vi "Dashboard Main.vi"() -> ()   [LabVIEW 2015]
uses:
  <vilib>/Utility/miscctls.llb/LVRowAndColumnTypeDef.ctl
  <vilib>/event_ctls.llb/eventvkey.ctl
  <vilib>/Rock Robotics/WPI/Dashboard/WPI_DashboardLogging Global.vi
  <vilib>/Rock Robotics/Network Tables/NT Read Numeric Array.vi
  <vilib>/Utility/config.llb/Write Key (String).vi
  <vilib>/Utility/config.llb/Write Key (I32).vi
  <vilib>/Utility/config.llb/NI_LVConfig.lvlib
panel:
  in  "Stop":bool
  in  "TCP":refnum<k5>
  in  "Rec Mode":enum32{"Stop", "Record", "Playback"}(radio)
  in  "Vision":u16(ring) items=["Camera Off", "USB Camera SW", "USB Camera HW", "IP Camera"]
  out "Camera IP":string
  out "Image Message":string="Timeout in Camera Communications"
  in  "Dashboard Tab":T1(tab)
  out "NT Connected":bool
  in  "Camera Settings":T2={"Frame Rate"=30, "Compression"=30, "Size"=1} {"Frame Rate" scale=1.0..30.0; "Size" items=["640x480", "320x240", "160x120"]}
  out "MotorChart R":cluster{"Numeric":dbl, "Numeric":dbl}(graph)
  out "MotorChart L":T3(graph)
  out "MotorSliders R":cluster{"MotorSlide1":dbl, "MotorSlide2":dbl} {"MotorSlide2" scale=-1.0..1.0 scale format="%#_2e"; "MotorSlide1" scale=-1.0..1.0 scale format="%#_2e"}
  out "MotorSliders L":T4 {"MotorSlide4 2" scale=0.0..14.0 scale format="%#_2e"; "MotorSlide2" scale=-1.0..1.0 scale format="%#_2e"; "MotorSlide1" scale=-1.0..1.0 scale format="%#_2e"}
  out "Gyro":dbl(knob) scale=0.0..360.0
  out "JS1 Z":dbl(slide) scale=-1.0..1.0 scale format="%#_2e"
  out "JS1 Graph":cluster{"X":dbl, "Y":dbl}[](graph)
  out "JS1 Buttons":T5
  out "JS2 Z":dbl(slide) scale=-1.0..1.0 scale format="%#_2e"
  out "JS2 Graph":cluster{"X":dbl, "Y":dbl}[](graph)
  out "JS2 Buttons":T5
  out "Mode":T6(ring)=enum."Auto Disabled"
  in  "DB Camera Config":bool
  out "fps":dbl format="%#.1g"
  out "Mbps":dbl format="%#.1g"
  out "Mbps 2":bool
  in  "DB/String 9":string
  in  "DB/String 8":string
  in  "DB/String 7":string
  in  "DB/String 6":string
  in  "DB/String 5":string
  in  "DB/String 4":string
  in  "DB/String 3":string
  in  "DB/String 2":string
  in  "DB/String 1":string
  in  "DB/String 0":string
  in  "DB/Slider 0":dbl(slide) scale=0.0..5.0
  in  "DB/Slider 1":dbl(slide) scale=0.0..5.0
  in  "DB/Slider 2":dbl(slide) scale=0.0..5.0
  in  "DB/Slider 3":dbl(slide) scale=0.0..5.0
  out "DB/LED 3":bool
  out "DB/LED 2":bool
  out "DB/LED 1":bool
  out "DB/LED 0":bool
  in  "DB/Button 3":bool
  in  "DB/Button 2":bool
  in  "DB/Button 1":bool
  in  "DB/Button 0":bool caption="New Name"
  out "Data AQ - Y axis":dbl(graph)
  out "Turn Power":dbl
  out "Throttle":dbl
  in  "Ka":dbl
  in  "Kv":dbl=0.08333
  in  "Max Acceleration":dbl=8.0
  in  "Max Velocity":dbl=13.5
  in  "Drive Distance":dbl
  in  "Test Slider":dbl(slide) scale=0.0..100.0 scale format="%#_3g"
  in  "On/Off":bool caption="Solenoid"
  in  "Test Name":u16(ring) items=["Select the test to run..."]
  in  "Test Tree":string(tree)
  in  "Motor":cluster{"Value":dbl, "Enable":bool} {"Value" scale=-1.0..1.0 scale format="%#_3g"}
  out "Progress":T7 {"Test Progress" scale=0.0..100.0}
  in  "Rev/Fwd":cluster{"Forward":bool, "Reverse":bool}
  in  "Test Ring":u16(ring) items=["Monochrome", "Color"]
  out "Cmd Status":string
  in  "Execute Command":bool
  in  "Command Params":string[][](table)
  in  "Command Selection":i32(listbox)
  in  "CheckList":i32(listbox)
  out "Tree":string(tree)
  out "Camera Image":T8(plugin-control)
  out "Boolean":bool
  # "Left"
  # "Front"
  # "Right"
  # "Battery"
  # "This tab is a great place for autonomous settings and robot-specific values.\nPlace controls and indicators inside this tab and match name to\nDashboard Variables on robot. You can also delete this comment."
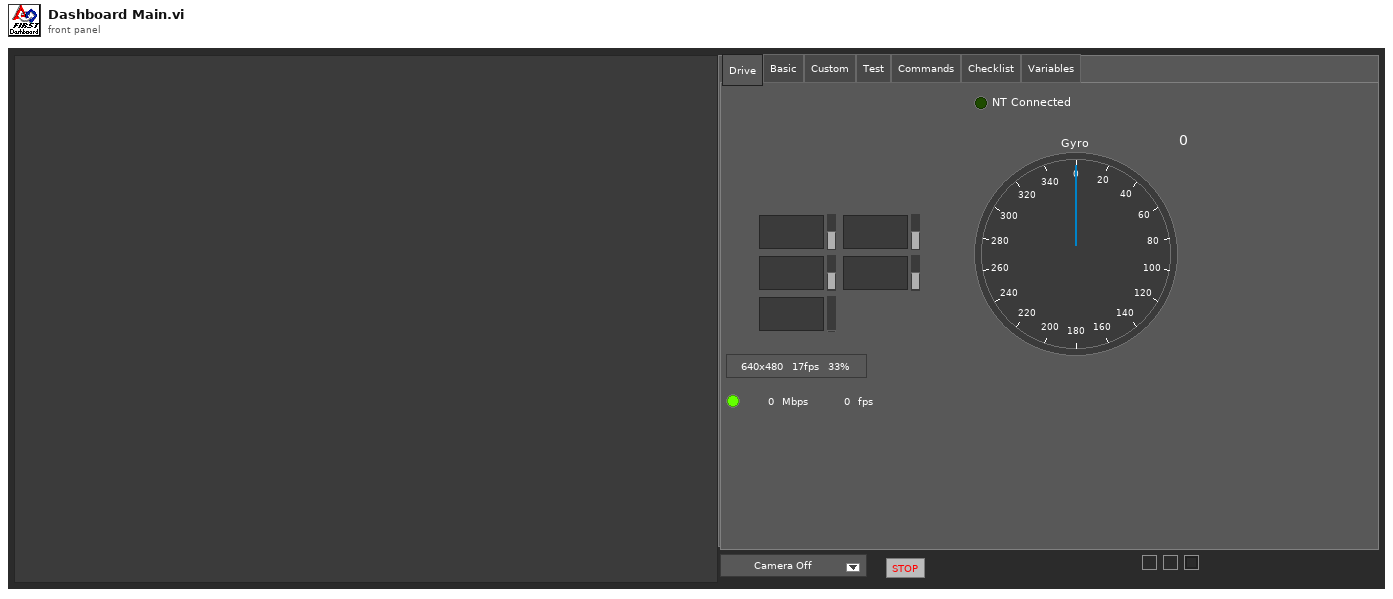
[diagram p1: front panel]
types:
  T1 = enum32{"Drive", "Basic", "Custom", "Test", "Commands", "Checklist", "Variables"}
  T2 = cluster{"Frame Rate":i32, "Compression":i32, "Size":u16}
  T3 = cluster{"Numeric":dbl, "Numeric":dbl, "Battery V":dbl}
  T4 = cluster{"MotorSlide1":dbl, "MotorSlide2":dbl, "MotorSlide4 2":dbl}
  T5 = cluster{bool, bool, bool, bool, bool, bool, bool, bool, bool, bool, bool, bool}
  T6 = enum8{"Tele-Op Disabled", "Tele-Op Enabled", "Auto Disabled", "Auto Enabled", "Test Disabled", "Test Enabled", "Disconnected", "No Code", "E-Stop"}
  T7 = cluster{"Test Progress":u8, "Test Progress Text":string}
  T8 = typedef "IMAQ Image.ctl" = refnum<image>
  T9 = cluster{"IDs":cluster{"RPC field ID":u16, "Unique ID":u16}, "String":string}
  T10 = enum32{"Drive", "Basic", "Custom", "Test", "Checklist", "Variables"}
  T11 = typedef "Image Type" = u32
  T12 = cluster{"Camera Image":refnum<vi>, "Dashboard Tab":refnum<vi>, "Boolean":refnum<vi>, "Vision":refnum<vi>, "Rec Mode":refnum<vi>, "Test Slider":refnum<vi>, "On/Off ":refnum<vi>, "Test Ring":refnum<vi>, "Rev/Fwd":refnum<vi>, "Test Name":refnum<vi>, "Motor":refnum<vi>, "Progress":refnum<vi>, "CheckList":refnum<vi>, "Tree":refnum<vi>, "Test Tree":refnum<vi>, "Command Params":refnum<vi>, "Command Selection":refnum<vi>, "Execute Command":refnum<vi>, "Cmd Status":refnum<vi>}
  T13 = cluster{"Error Strings":string, "Disable Counts":cluster{u16, u16}, "Rail Faults":cluster{u16, u16, u16}, "Robot IP":string, "DB Mode":u8, "Event Info":cluster{"Name":string, "Type":u8, "Number":u16, "Replay":u8}, "Camera Addr":string}
  T14 = cluster{"Storage":cluster{"Disk Free":u64, "RAM Block":u32, "RAM free":u32}, "CPU Utilization":cluster{"CPU % ISR":sgl, "CPU % Time Crit":sgl, "CPU % Timed Str":sgl, "CPU % High":sgl, "CPU % Above":sgl, "CPU % Normal":sgl, "CPU % Low":sgl}, "CAN":cluster{"% Bus Utilization":sgl, "Bus Off Cnt":u32, "TX_FIFO Full Cnt":u32, "Receive Error Cnt":u8, "Transmit Error Cnt":u8}, "HID":cluster{"HID Outputs":u32, "Rumble Low":u16, "Rumble High":u16}[]}
  T15 = cluster{"Status bits":cluster{"Test Mode":bool, "Autonomous":bool, "Enabled":bool, "Code Start":bool, "Brownout":bool, "Reserved 2":bool, "Reserved 3":bool, "E-Stop":bool}, "Code Trace":cluster{"Disabled":bool, "TeleOp":bool, "Auto":bool, "Test":bool}, "Controller Type":enum16{"unknown", "cRIO", "roboRio"}, "Code?":enum16{"unknown", "noCode", "code"}, "Battery V":dbl}
  T16 = cluster{"Control Bits":cluster{"TestMode":bool, "Autonomous":bool, "Enabled":bool, "FMS Present":bool, bool, bool, bool, "E-Stop":bool}, "Team Station ":u8, "Countdown":sgl, "Joystick Values":cluster{"Axes":dbl[], "Buttons":bool[], "POVs":i16[]}[]}
  T17 = cluster{"Axes":dbl[], "Buttons":bool[], "POVs":i16[]}[]
  T18 = cluster{"Axes":dbl[], "Buttons":bool[], "POVs":i16[]}
  T19 = cluster{"Buttons[0]":bool, "Buttons[1]":bool, "Buttons[2]":bool, "Buttons[3]":bool, "Buttons[4]":bool, "Buttons[5]":bool, "Buttons[6]":bool, "Buttons[7]":bool, "Buttons[8]":bool, "Buttons[9]":bool, "Buttons[10]":bool, "Buttons[11]":bool}
  T20 = typedef "NI_LVConfig.lvlib/Config Data RefNum.ctl" = refnum<k1>
  T21 = cluster{"Operation":enum16{"Update", "Clear"}, "Color Box":u32}[]
  T22 = typedef "eventvkey.ctl" = enum16{"ASCII", "Enter", "Return", "Shift", "Ctrl", "Alt", "Cmd", "Opt", "Caps", "NumLock", "Clear", "Break", "Up", "Down", "Left", "Right", "Insert", "Delete", "Home", "End", "PageUp", "PageDown", "Escape", "Help", "Pause", "ScrollLock", "F1", "F2", "F3", "F4", "F5", "F6", "F7", "F8", "F9", "F10", "F11", "F12", "F13", "F14", "F15", "F16", "F17", "F18", "F19", "F20", "F21", "F22", "F23", "F24", "Play", "VolumeUp", "VolumeDown", "Mute", "Two Byte Char"}
  T23 = cluster{"Image Size":bool, "Image Type":bool, "Pixel Value":bool, "ROI Information":bool, "Zoom Factor":bool}
  T24 = enum8{"Enabled", "Disabled", "Disabled and Grayed Out"}
  T25 = cluster{"Operation":enum16{"Update", "Clear"}, "Color Box":u32}
  T26 = typedef "LVRowAndColumnTypeDef.ctl" = cluster{"Row":i32, "Column":i32}
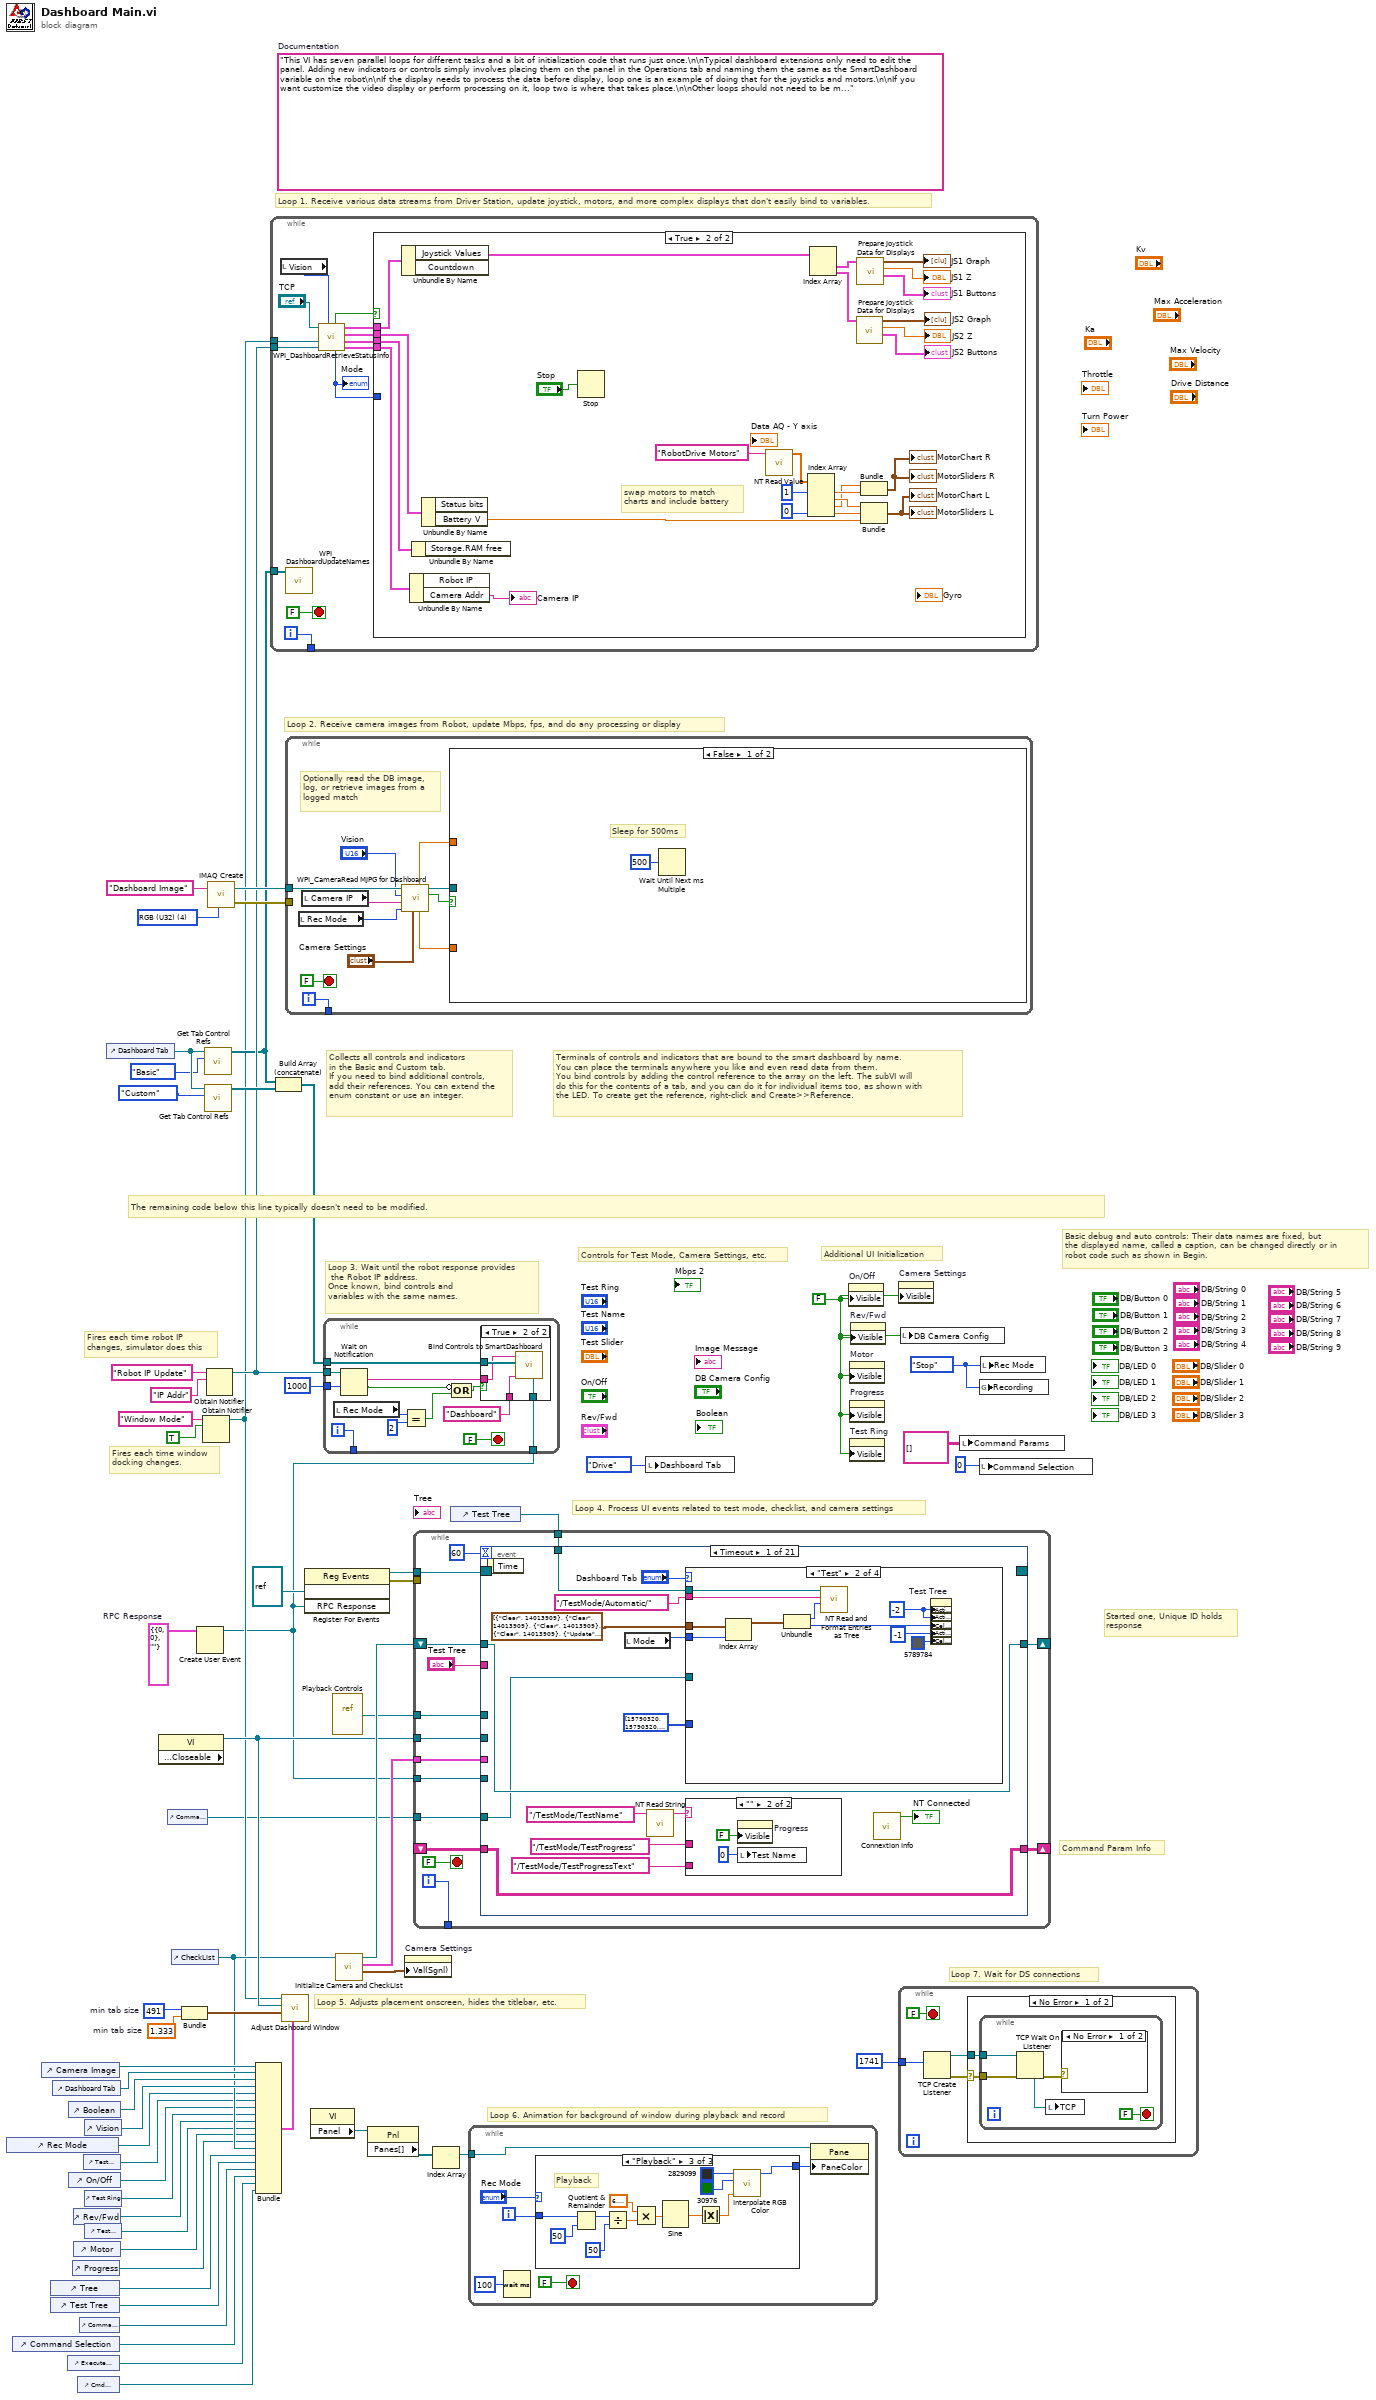
[diagram p0: block diagram]
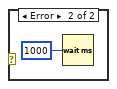
[diagram p2: hidden frame]
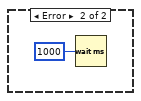
[diagram p3: hidden frame]
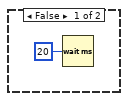
[diagram p4: hidden frame]
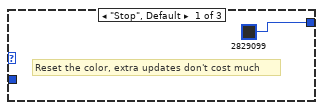
[diagram p5: hidden frame]
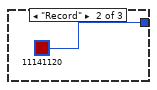
[diagram p6: hidden frame]
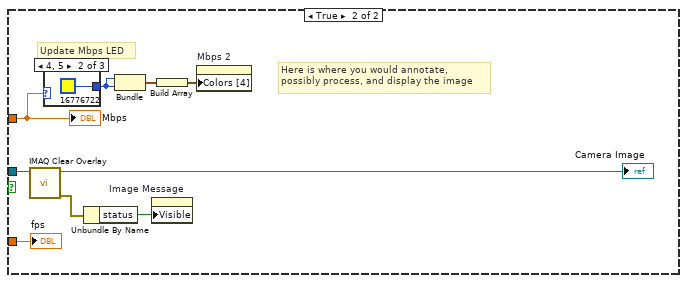
[diagram p8: hidden frame]
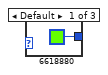
[diagram p9: hidden frame]
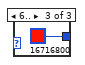
[diagram p10: hidden frame]
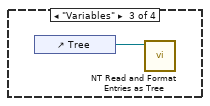
[diagram p12: hidden frame]
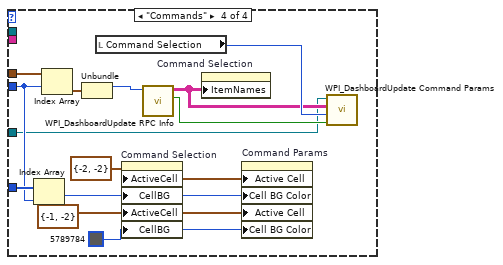
[diagram p13: hidden frame]
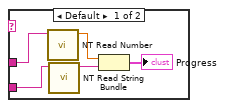
[diagram p14: hidden frame]
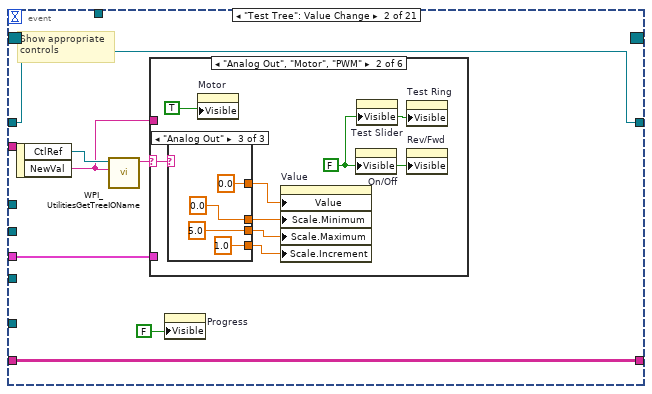
[diagram p15: hidden frame]
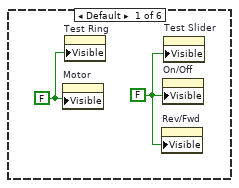
[diagram p16: hidden frame]
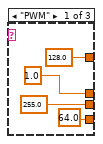
[diagram p17: hidden frame]
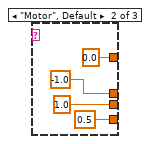
[diagram p18: hidden frame]
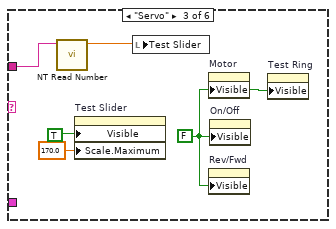
[diagram p19: hidden frame]
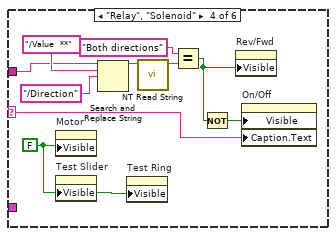
[diagram p20: hidden frame]
diagram:
  w7 = T9 {"IDs"={"RPC field ID"=0, "Unique ID"=0}, "String"=""}  # RPC Response
  w33 = 491  # min tab size
  w32 = 1.333  # min tab size
  w41 = enum32{"Stop", "Record", "Playback"}."Stop" ("Rec Mode")
  w15 = FALSE ("Visible")
  (unwired) "This VI has seven parallel loops for different tasks and a bit of initialization code that runs just once.\n\nTypical dashboard extensions only need to edit the panel. Adding new indicators or controls simply involves placing them on the panel in the Operations tab and naming them the same as the SmartDashboard variable on the robot\n\nIf the display needs to process the data before display, loop one is an example of doing that for the joysticks and motors.\n\nIf you want customize the video display or perform processing on it, loop two is where that takes place.\n\nOther loops should not need to be modified. They are pretty standard, and document the task they perform."  # Documentation
  w61 = T11 4 items=["Grayscale (U8)", "Grayscale (I16)", "Grayscale (SGL)", "Complex (CSG)", "RGB (U32)", "HSL (U32)", "RGB (U64)"] ("Image Type")
  # "Command Param Info"
  # "Started one, Unique ID holds\nresponse"
  # "Loop 7. Wait for DS connections"
  # "Basic debug and auto controls: Their data names are fixed, but\nthe displayed name, called a caption, can be changed directly or in\nrobot code such as shown in Begin."
  # "Controls for Test Mode, Camera Settings, etc."
  # "Additional UI Initialization"
  # "Loop 6. Animation for background of window during playback and record"
  # "Fires each time robot IP\nchanges, simulator does this"
  # "Fires each time window\ndocking changes."
  # "Collects all controls and indicators\nin the Basic and Custom tab.\nIf you need to bind additional controls,\nadd their references. You can extend the\nenum constant or use an integer."
  # "The remaining code below this line typically doesn't need to be modified."
  # "Loop 4. Process UI events related to test mode, checklist, and camera settings"
  # "Terminals of controls and indicators that are bound to the smart dashboard by name.\nYou can place the terminals anywhere you like and even read data from them.\nYou bind controls by adding the control reference to the array on the left. The subVI will\ndo this for the contents of a tab, and you can do it for individual items too, as shown with\nthe LED. To create get the reference, right-click and Create>>Reference."
  # "Loop 3. Wait until the robot response provides\n the Robot IP address.\nOnce known, bind controls and\nvariables with the same names."
  # "Loop 5. Adjusts placement onscreen, hides the titlebar, etc."
  # "Loop 1. Receive various data streams from Driver Station, update joystick, motors, and more complex displays that don't easily bind to variables."
  # "Loop 2. Receive camera images from Robot, update Mbps, fps, and do any processing or display"
  n1 = control-ref of="Rec Mode"() -> (w21:refnum<vi>)
  n2 = control-ref of="Command Selection"() -> (w6:refnum<vi>)
  n3 = control-ref of="Camera Image"() -> (w36:refnum<vi>)
  n4 = control-ref of="Tree"() -> (w25:refnum<vi>)
  n5 = control-ref of="Test Tree"() -> (w24:refnum<vi>)
  n6 = control-ref of="Dashboard Tab"() -> (w35:refnum<vi>)
  n7 = control-ref of="Execute Command"() -> (w8:refnum<vi>)
  n8 = control-ref of="Boolean"() -> (w30:refnum<vi>)
  n9 = control-ref of="On/Off"() -> (w19:refnum<vi>)
  n10 = control-ref of="Progress"() -> (w16:refnum<vi>)
  n11 = control-ref of="Rev/Fwd"() -> (w17:refnum<vi>)
  n12 = control-ref of="Motor"() -> (w22:refnum<vi>)
  n13 = control-ref of="Cmd Status"() -> (w2:refnum<vi>)
  n14 = control-ref of="Command Params"() -> (w9:refnum<vi>)
  n15 = control-ref of="Test Slider"() -> (w20:refnum<vi>)
  n16 = control-ref of="Vision"() -> (w34:refnum<vi>)
  n17 = control-ref of="Test Ring"() -> (w18:refnum<vi>)
  n18 = control-ref of="Test Name"() -> (w23:refnum<vi>)
  n19 = control-ref of="Dashboard Tab"() -> (w39:refnum<vi>)
  n20 = property class="VI" props=["Front Panel.Closeable"]() -> (reference out=w40:refnum<vi>)  [unwired: 2 in, 2 out]
  n21 = control-ref of="Command Params"() -> (w1:refnum<vi>)
  n22 = control-ref of="CheckList"() -> (w26:refnum<vi>)
  n23 = Bundle("min tab size"=w33, "min tab size"=w32) -> (w31:cluster{"min tab size":i32, "min tab size":dbl})  [unwired: 1 in]
  n24 = Create User Event(user event datatype=w7) -> (user event=w3:refnum<user-event>)  [unwired: 1 in, 1 out]
  n25 = Obtain Notifier(name (unnamed)="Window Mode", notification data type=TRUE) -> (notifier out=w12:refnum<notifier>)  [unwired: 2 in, 2 out]
  n26 = call <vilib>:"Get Tab Control Refs.vi"("Page Index"=T10."Basic" ("Dashboard Tab"), "TabControl in"=w39) -> ("ControlsOnPage"=w13:refnum<vi>[])  [unwired: 9 in]
  n27 = call <vilib>:"Get Tab Control Refs.vi"("Page Index"=T10."Custom" ("Dashboard Tab"), "TabControl in"=w39) -> ("ControlsOnPage"=w38:refnum<vi>[])  [unwired: 9 in]
  n28 = Obtain Notifier(name (unnamed)="Robot IP Update", notification data type="IP Addr" ("name (unnamed)")) -> (notifier out=w14:refnum<notifier>)  [unwired: 2 in, 2 out]
  n29 = call "IMAQ Create"("Image Name"="Dashboard Image", "Image Type"=w61) -> ("New Image"=w59:T8, "error out"=w58:errorcluster)  [unwired: 2 in, 1 out]
  n30 = Bundle("Camera Image"=w36, "Dashboard Tab"=w35, "Boolean"=w30, "Vision"=w34, "Rec Mode"=w21, "Test Slider"=w20, "On/Off"=w19, "Test Ring"=w18, "Rev/Fwd"=w17, "Test Name"=w23, "Motor"=w22, "Progress"=w16, "CheckList"=w26, "Tree"=w25, "Test Tree"=w24, "Command Params"=w9, "Command Selection"=w6, "Execute Command"=w8, "Cmd Status"=w2) -> (w27:T12)  [unwired: 1 in]
  n31 = while {
    tunnel: [w73] -> _
    tunnel: w14 -> [w67]
    tunnel: w13 -> [w66]
    tunnel: w12 -> [w62]
    i -> [w73]
    stop <- FALSE stop-if-true
    n32 = local read "Vision"() -> (w64:u16)
    n33 = call <vilib>:"WPI_DashboardUpdateNames.vi"("Controls on Tab"=w66) -> ()  [unwired: 11 in]
    n34 = call <vilib>:"WPI_DashboardRetrieveStatusInfo.vi"("Vision"=w64, "Binding Refnum"=w67, "Window Mode Notifier"=w62, "TCP Cnx"="TCP") -> ("Power and Errors"=w68:T13, "Robot Metrics"=w71:T14, "Status Info"=w72:T15, "Control Info"=w69:T16, "Robot Mode"=w65:T6, "Process?"=w70:bool)  [unwired: 2 in]
    "Mode" <- w65
    n35 = case shown="True" w70 {
      tunnel: w72 -> [_ w101]
      tunnel: w71 -> [_ w100]
      tunnel: w69 -> [_ w99]
      tunnel: w68 -> [_ w98]
      tunnel: w65 -> [_ _]
      frame False {
        n36 = Wait (ms)(milliseconds to wait=u32 20) -> ()  [unwired: 1 out]
      }
      frame True {
        # "swap motors to match\ncharts and include battery"
        n37 = Unbundle By Name(w99) -> ("Joystick Values"=w88:T17)  [unwired: 1 out]
        n38 = Unbundle By Name(w98) -> ("Camera Addr"=→"Camera IP":string)  [unwired: 1 out]
        n39 = Unbundle By Name(w100) -> ()  [unwired: 1 out]
        n40 = Unbundle By Name(w101) -> ("Battery V"=w89:dbl)  [unwired: 1 out]
        n41 = Stop(stop? (T)="Stop") -> ()
        n42 = call-poly <vilib>:"NT Read Value.vi"("Name"="RobotDrive Motors") -> ("Numeric Array"=w77:dbl[])  [unwired: 9 in, 1 out]
        n43 = Index Array(array=w77, index #1=1, index #4=0) -> (element #1=w93:dbl, element #2=w94:dbl, element #3=w92:dbl, element #4=w97:dbl)  [unwired: 2 in]
        n44 = Index Array(array=w88) -> (element #1=w87:T18, element #2=w82:T18)  [unwired: 2 in]
        n45 = call "Prepare Joystick Data for Displays.vi"("Joystick Values"=w82) -> ("Buttons"=→"JS2 Buttons":T19, "Z Axis"=→"JS2 Z":dbl, "Cartesian Data"=→"JS2 Graph":cluster{"X axis":dbl, "X axis":dbl}[])  [unwired: 8 in]
        n46 = call "Prepare Joystick Data for Displays.vi"("Joystick Values"=w87) -> ("Buttons"=→"JS1 Buttons":T19, "Z Axis"=→"JS1 Z":dbl, "Cartesian Data"=→"JS1 Graph":cluster{"X axis":dbl, "X axis":dbl}[])  [unwired: 8 in]
        n47 = Bundle("Numeric"=w92, "Numeric"=w93) -> (→"MotorChart R" →"MotorSliders R":cluster{"Numeric":dbl, "Numeric":dbl})  [unwired: 1 in]
        n48 = Bundle("Numeric"=w94, "Numeric"=w97, "Battery V"=w89) -> (→"MotorChart L" →"MotorSliders L":T3)  [unwired: 1 in]
      }
    }
  }
  n49 = Build Array (concatenate)(w13, w38) -> (w37:refnum<vi>[])
  n50 = call "Adjust Dashboard Window.vi"("Sizing Refnums"=w27, "Size Constraints"=w31, "VI"=w40, "WIn Mode"=w12) -> ()  [unwired: 8 in]
  n51 = while {
    tunnel: w59 -> [w110]
    tunnel: w58 -> [_]
    tunnel: [w111] -> _
    i -> [w111]
    stop <- FALSE stop-if-true
    # "Optionally read the DB image,\nlog, or retrieve images from a\nlogged match"
    n52 = local read "Rec Mode"() -> (w104:enum32{"Stop", "Record", "Playback"})
    n53 = local read "Camera IP"() -> (w102:string)
    n54 = call <vilib>:"WPI_CameraRead MJPG for Dashboard.vi"("Camera Settings"="Camera Settings", "Rec Mode"=w104, "Camera IP"=w102, "Camera Mode"="Vision", "Refnum in"=w110) -> ("Active"=w108:bool, "Refnum out"=w109:T8, "FPS"=w107:dbl, "Bandwidth (Mbps)"=w106:dbl)  [unwired: 3 in]
    n55 = case shown="False" w108 {
      tunnel: w109 -> [_ w117]
      tunnel: w106 -> [_ w116]
      tunnel: w107 -> [_ w114]
      frame False {
        # "Sleep for 500ms"
        n56 = Wait Until Next ms Multiple(millisecond multiple=u32 500) -> ()  [unwired: 1 out]
      }
      frame True {
        # "Here is where you would annotate,\npossibly process, and display the image"
        # "Update Mbps LED"
        n57 = call "IMAQ Clear Overlay"("Image"=w117) -> ("error out"=w121:errorcluster, "Image Out"=→"Camera Image":T8)  [unwired: 2 in, 7 out]
        n58 = case shown="4, 5" w116 {
          tunnel: [u32 6618880 ("Color Box") u32 16776722 ("Color Box") u32 16716800 ("Color Box")] -> w118
          frame Default {
          }
          frame 4, 5 {
          }
          frame 6.. {
          }
        }
        n59 = Unbundle By Name(w121) -> ("status"=w122:bool)
        n60 = Bundle("Color Box"=w118, "Color Box"=w118) -> (w120:cluster{"Color Box":u32, "Color Box":u32})  [unwired: 1 out]
        n61 = property on="Image Message" class="Str"("Visible"=w122) -> ()  [unwired: 2 in, 2 out]
        n62 = Build Array(w120) -> (w119:cluster{"Color Box":u32, "Color Box":u32}[])
        n63 = property on="Mbps 2" class="Bool (strict)"("Colors [4]"=w119) -> ()  [unwired: 2 in, 2 out]
        "Mbps" <- w116
        "fps" <- w114
      }
    }
  }
  n64 = register-events(refnum<vi> refnum, w3) -> (reference out=w45:refnum<event-registration>, error out=w44:errorcluster)  [unwired: 2 in]
  n65 = property class="VI"() -> ("Panel"=w48:refnum<vi>)  [unwired: 2 in, 2 out]
  n66 = while {
    tunnel: w37 -> [w138]
    tunnel: w14 -> [w136]
    tunnel: [w134] -> _
    tunnel: u32 1000 ("milliseconds to wait") -> [w133]
    tunnel: w3 -> [w126]
    i -> [w134]
    stop <- FALSE stop-if-true
    n67 = local read "Rec Mode"() -> (w129:enum32{"Stop", "Record", "Playback"})
    n68 = Wait on Notification(notifier=w136, timeout in ms (-1)=w133) -> (notification=w135:string, timed out?=w131:bool)  [unwired: 2 in, 2 out]
    n69 = Equal?(x=w129, y=u16 2 ("Rec Mode")) -> (x = y?=w130:bool)
    n70 = Compound Arithmetic op=OR(invert w131, w130) -> (w132:bool)
    n71 = case shown="True" w132 {
      tunnel: w138 -> [_ w142]
      tunnel: w135 -> [_ w141]
      tunnel: "Dashboard" -> [_ w140]
      tunnel: w126 -> [_ w139]
      frame False {
      }
      frame True {
        n72 = call <vilib>:"Bind Controls to SmartDashboard.vi"("RPC ref"=w139, "Client Name"=w140, "Bound Control Refs"=w142, "Server IP Address"=w141) -> ()  [unwired: 8 in]
      }
    }
  }
  n73 = vi-ref "Playback Controls.vi"() -> (w46:refnum<vi>)
  n74 = call "Initialize Camera and CheckList.vi"("ListBox in"=w26) -> ("Cluster"=w52:cluster{"value":i32, "value":i32, "index":i32}, "Array"=w53:cluster{string[]}[], "File Refnum"=w51:T20)  [unwired: 8 in]
  n75 = property class="Pnl"(reference=w48) -> ("Panes[]"=w49:refnum<vi>[])  [unwired: 1 in, 2 out]
  n76 = property on="Camera Settings" class="Clust (strict)"("Val(Sgnl)"=w52) -> ()  [unwired: 2 in, 2 out]
  n77 = Index Array(array=w49) -> (element=w47:refnum<vi>)  [unwired: 1 in]
  n78 = control-ref of="Test Tree"() -> (w50:refnum<vi>)
  n79 = while {
    tunnel: w53 -> [w154]
    shift-right: [w153] -> _
    shift-left: w51 -> [w152]
    tunnel: [w151] -> _
    tunnel: w50 -> [w150]
    tunnel: w46 -> [w149]
    tunnel: w45 -> [w148]
    tunnel: w44 -> [_]
    tunnel: w40 -> [w147]
    tunnel: w3 -> [w146]
    tunnel: w1 -> [w145]
    shift-right: [w144] -> _
    shift-left: _ -> [w143]
    i -> [w151]
    stop <- FALSE stop-if-true
    n80 = event shown="[0] Timeout" {
      selector: w148 -> [_ _ _ _ _ _ _ _ _ _ _ _ _ _ _ _ _ _ _ _ _]
      dyn-events: [_ _ _ _ _ _ _ _ _ _ _ _ _ _ _ _ w455 _ _ _ _] -> _
      timeout: u32 60 ("milliseconds to wait") -> [_ _ _ _ _ _ _ _ _ _ _ _ _ _ _ _ _ _ _ _ _]
      tunnel: w150 -> [w167 _ _ _ _ _ _ _ _ _ _ _ _ _ _ _ _ _ _ _ _]
      tunnel: "Test Tree" -> [_ _ _ _ _ _ _ _ _ _ _ w418 w427 w430 w435 w444 _ _ _ _ _]
      tunnel: w154 -> [_ w205 _ _ _ _ _ _ _ w380 w411 _ _ _ _ _ _ _ _ _ _]
      tunnel: [w164 w204 w308 w314 w326 w338 w346 w352 w365 w379 w404 w417 w425 w429 w434 w443 w457 w473 w475 w483 w494] -> w153
      tunnel: w152 -> [w164 w204 w308 w314 w326 w338 w346 w352 w365 w378 w404 w417 w425 w429 w434 w443 w457 w473 w475 w483 w494]
      tunnel: w149 -> [_ _ _ _ _ _ _ _ _ _ _ _ _ _ _ _ w458 _ w478 _ _]
      tunnel: w147 -> [_ _ _ _ _ _ _ _ _ _ _ _ _ _ _ _ w453 _ _ _ _]
      tunnel: w146 -> [_ _ _ _ _ _ _ _ _ _ _ _ _ _ _ _ w449 _ _ _ _]
      tunnel: w145 -> [w159 _ _ _ w324 _ _ _ _ _ _ _ _ _ _ _ _ _ _ _ _]
      tunnel: [w158 w203 w307 w313 w322 w332 w343 w351 w364 w377 w403 w416 w424 w428 w433 w442 w448 w471 w474 w479 w487] -> w144
      tunnel: w143 -> [w158 w203 w307 w313 w322 _ _ w351 w364 w377 w403 w416 w424 w428 w433 w442 w448 w471 w474 w479 w487]
      event Timeout {
        n81 = event-data() -> ()  [unwired: 1 in, 1 out]
        n82 = local read "Mode"() -> (w161:T6)
        n83 = call <vilib>:"NT Read String.vi"("Name"="/TestMode/TestName") -> ("String"=w170:string)  [unwired: 9 in, 1 out]
        n84 = case shown="\"Test\"" "Dashboard Tab" {
          tunnel: w167 -> [_ w181 _ _]
          tunnel: "/TestMode/Automatic/" ("Name Pattern") -> [_ w180 _ _]
          tunnel: T21 [{"Operation"=enum."Clear", "Color Box"=14013909}, {"Operation"=enum."Clear", "Color Box"=14013909}, {"Operation"=enum."Clear", "Color Box"=14013909}, {"Operation"=enum."Clear", "Color Box"=14013909}, {"Operation"=enum."Update", "Color Box"=14013909}, {"Operation"=enum."Update", "Color Box"=16777215}, {"Operation"=enum."Clear", "Color Box"=14013909}, {"Operation"=enum."Clear", "Color Box"=14013909}, {"Operation"=enum."Clear", "Color Box"=14013909}] -> [_ w173 _ w190]
          tunnel: w161 -> [_ w172 _ w189]
          tunnel: u32[] [15790320, 15790320, 15790320, 15790320, 16777215, 16777215, 15790320, 15790320, 15790320] -> [_ _ _ w195]
          tunnel: w159 -> [_ _ _ w183]
          frame "Custom", Default {
          }
          frame "Test" {
            w179 = -2 ("Active Item:Row Number")
            n85 = Index Array(array=w173, index=w172) -> (element=w174:T25)
            n86 = Unbundle(w174) -> ("Operation"=w175:enum16{"Update", "Clear"}, "Color Box"=w176:u32)
            n87 = call <vilib>:"NT Read and Format Entries as Tree.vi"("Operation"=w175, "Name Pattern"=w180, "Tree Refnum"=w181) -> ()  [unwired: 7 in, 2 out]
            n88 = property on="Test Tree" class="Tree (strict)"("Active Item Row Number"=w179, "ActiveColNum"=w179, "CellBG"=w176, "Active Item Row Number"=-1 ("Active Item:Row Number"), "CellBG"=u32 5789784 ("Color Box")) -> ()  [unwired: 2 in, 2 out]
          }
          frame "Variables" {
            n89 = control-ref of="Tree"() -> (w182:refnum<vi>)
            n90 = call <vilib>:"NT Read and Format Entries as Tree.vi"("Tree Refnum"=w182) -> ()  [unwired: 9 in, 2 out]
          }
          frame "Commands" {
            w191 = u32 5789784 ("Color Box")
            w192 = T26 {"Row"=-1, "Column"=-2} ("Active Cell:Active Cell")
            w194 = T26 {"Row"=-2, "Column"=-2} ("Active Cell:Active Cell")
            n91 = Index Array(array=w195, index=w189) -> (element=w193:u32)
            n92 = Index Array(array=w190, index=w189) -> (element=w188:T25)
            n93 = Unbundle(w188) -> ("Operation"=w187:enum16{"Update", "Clear"})  [unwired: 1 out]
            n94 = local read "Command Selection"() -> (w186:i32)
            n95 = property on="Command Selection" class="MCListbox (strict)"("ActiveCell"=w194, "CellBG"=w193, "ActiveCell"=w192, "CellBG"=w191) -> ()  [unwired: 2 in, 2 out]
            n96 = call <vilib>:"WPI_DashboardUpdate RPC Info.vi"("Operation"=w187) -> ("update"=w185:bool, "commands"=w184:string[][])  [unwired: 9 in]
            n97 = property on="Command Selection" class="MCListbox (strict)"("ItemNames"=w184) -> ()  [unwired: 2 in, 2 out]
            n98 = property on="Command Params" class="Tbl (strict)"("Active Cell"=w194, "Cell BG Color"=w193, "Active Cell"=w192, "Cell BG Color"=w191) -> ()  [unwired: 2 in, 2 out]
            n99 = call <vilib>:"WPI_DashboardUpdate Command Params.vi"("Update"=w185, "NewVal"=w186, "Commands"=w184, "Param Tbl"=w183) -> ()  [unwired: 7 in, 1 out]
          }
        }
        n100 = case shown="\"\"" w170 {
          tunnel: "/TestMode/TestProgress" ("Name") -> [w197 _]
          tunnel: "/TestMode/TestProgressText" ("Name") -> [w196 _]
          frame Default {
            n101 = call <vilib>:"NT Read Number.vi"("Name"=w197) -> ("Numeric"=w198:dbl)  [unwired: 9 in, 1 out]
            n102 = call <vilib>:"NT Read String.vi"("Name"=w196) -> ("String"=w199:string)  [unwired: 9 in, 1 out]
            n103 = Bundle("Numeric"=w198, "String"=w199) -> (→"Progress":cluster{"Numeric":dbl, "String":string})  [unwired: 1 in]
          }
          frame "" {
            n104 = property on="Progress" class="Clust (strict)"("Visible"=FALSE) -> ()  [unwired: 2 in, 2 out]
            n105 = local write "Test Name"(u16 0) -> ()
          }
        }
        n106 = call <vilib>:"Connextion Info.vi"() -> ("Connected"=→"NT Connected":bool)  [unwired: 10 in, 1 out]
      }
      event "Test Tree": Value Change {
        # "Show appropriate\ncontrols"
        n107 = event-data() -> ("CtlRef"=w208:refnum<vi>, "NewVal"=w206:string)  [unwired: 1 in]
        n108 = call <vilib>:"WPI_UtilitiesGetTreeIOName.vi"("NewVal"=w206, "TreeControl in"=w208) -> ("I/O Name"=w209:string)  [unwired: 9 in]
        n109 = case shown="\"Analog Out\", \"Motor\", \"PWM\"" w209 {
          selector: w209 -> [_ w216 _ w238 w247 _]
          tunnel: w206 -> [_ _ w235 w237 _ w254]
          tunnel: w205 -> [_ _ _ _ _ w253]
          frame Default {
            w211 = FALSE ("Visible")
            w210 = FALSE ("Visible")
            n110 = property on="Motor" class="Clust (strict)"("Visible"=w210) -> ()  [unwired: 2 in, 2 out]
            n111 = property on="Test Ring" class="Ring (strict)"("Visible"=w210) -> ()  [unwired: 2 in, 2 out]
            n112 = property on="Rev/Fwd" class="Clust (strict)"("Visible"=w211) -> ()  [unwired: 2 in, 2 out]
            n113 = property on="On/Off" class="Bool (strict)"("Visible"=w211) -> ()  [unwired: 2 in, 2 out]
            n114 = property on="Test Slider" class="Slide (strict)"("Visible"=w211) -> ()  [unwired: 2 in, 2 out]
          }
          frame "Analog Out", "Motor", "PWM" {
            w217 = FALSE ("Visible")
            n115 = case shown="\"Analog Out\"" w216 {
              tunnel: [1.0 ("Value") -1.0 ("Value") 0.0 ("Value")] -> w215
              tunnel: [255.0 ("Value") 1.0 ("Value") 5.0 ("Value")] -> w214
              tunnel: [128.0 ("Value") 0.0 ("Value") 0.0 ("Value")] -> w213
              tunnel: [64.0 ("Value") 0.5 ("Value") 1.0 ("Value")] -> w212
              frame "PWM" {
              }
              frame "Motor", Default {
              }
              frame "Analog Out" {
              }
            }
            n116 = property on="Motor" class="Clust (strict)"("Visible"=TRUE) -> ()  [unwired: 2 in, 2 out]
            n117 = property on="Value" class="Slide (strict)"("Value"=w213, "Scale.Minimum"=w215, "Scale.Maximum"=w214, "Scale.Increment"=w212) -> ()  [unwired: 2 in, 2 out]
            n118 = property on="On/Off" class="Bool (strict)"("Visible"=w217) -> ()  [unwired: 2 in, 2 out]
            n119 = property on="Test Slider" class="Slide (strict)"("Visible"=w217) -> ()  [unwired: 2 in, 2 out]
            n120 = property on="Test Ring" class="Ring (strict)"("Visible"=w217) -> ()  [unwired: 2 in, 2 out]
            n121 = property on="Rev/Fwd" class="Clust (strict)"("Visible"=w217) -> ()  [unwired: 2 in, 2 out]
          }
          frame "Servo" {
            w233 = FALSE ("Visible")
            n122 = call <vilib>:"NT Read Number.vi"("Name"=w235) -> ("Numeric"=w234:dbl)  [unwired: 9 in, 1 out]
            n123 = property on="Test Slider" class="Slide (strict)"("Visible"=TRUE, "Scale.Maximum"=170.0 ("Scale.Range:Maximum")) -> ()  [unwired: 2 in, 2 out]
            n124 = local write "Test Slider"(w234) -> ()
            n125 = property on="Motor" class="Clust (strict)"("Visible"=w233) -> ()  [unwired: 2 in, 2 out]
            n126 = property on="Rev/Fwd" class="Clust (strict)"("Visible"=w233) -> ()  [unwired: 2 in, 2 out]
            n127 = property on="On/Off" class="Bool (strict)"("Visible"=w233) -> ()  [unwired: 2 in, 2 out]
            n128 = property on="Test Ring" class="Ring (strict)"("Visible"=w233) -> ()  [unwired: 2 in, 2 out]
          }
          frame "Relay", "Solenoid" {
            w236 = FALSE ("Visible")
            n129 = property on="Motor" class="Clust (strict)"("Visible"=w236) -> ()  [unwired: 2 in, 2 out]
            n130 = property on="Test Slider" class="Slide (strict)"("Visible"=w236) -> ()  [unwired: 2 in, 2 out]
            n131 = Search and Replace String(input string=w237, search string="/Value  **", replace string="/Direction") -> (result string=w243:string)  [unwired: 5 in, 3 out]
            n132 = property on="Test Ring" class="Ring (strict)"("Visible"=w236) -> ()  [unwired: 2 in, 2 out]
            n133 = call <vilib>:"NT Read String.vi"("Name"=w243) -> ("String"=w241:string)  [unwired: 9 in, 1 out]
            n134 = Equal?(x="Both directions", y=w241) -> (x = y?=w239:bool)
            n135 = Not(x=w239) -> (.not. x?=w240:bool)
            n136 = property on="Rev/Fwd" class="Clust (strict)"("Visible"=w239) -> ()  [unwired: 2 in, 2 out]
            n137 = property on="On/Off" class="Bool (strict)"("Visible"=w240, "Caption.Text"=w238) -> ()  [unwired: 2 in, 2 out]
          }
          frame "Compressor", "Digital Out" {
            w246 = FALSE ("Visible")
            # "Get direction and finish"
            n138 = property on="Motor" class="Clust (strict)"("Visible"=w246) -> ()  [unwired: 2 in, 2 out]
            n139 = property on="Test Slider" class="Slide (strict)"("Visible"=w246) -> ()  [unwired: 2 in, 2 out]
            n140 = property on="Test Ring" class="Ring (strict)"("Visible"=w246) -> ()  [unwired: 2 in, 2 out]
            n141 = property on="On/Off" class="Bool (strict)"("Visible"=TRUE, "Caption.Text"=w247) -> ()  [unwired: 2 in, 2 out]
            n142 = property on="Rev/Fwd" class="Clust (strict)"("Visible"=FALSE) -> ()  [unwired: 2 in, 2 out]
          }
          frame "Camera" {
            n143 = call <vilib>:"Get Last Path Segment.vi"("String in"=w254) -> ("String out"=w255:string)  [unwired: 10 in]
            n144 = property on="On/Off" class="Bool (strict)"("Visible"=FALSE) -> ()  [unwired: 2 in, 2 out]
            n145 = property on="Motor" class="Clust (strict)"("Visible"=FALSE) -> ()  [unwired: 2 in, 2 out]
            n146 = property on="Rev/Fwd" class="Clust (strict)"("Visible"=FALSE) -> ()  [unwired: 2 in, 2 out]
            n147 = case shown="\"White Balance  **\"" w255 {
              tunnel: w254 -> [w261 w270 w279 w288 w297 _ w303]
              tunnel: w253 -> [w259 w267 w276 w285 w294 _ _]
              frame "Size  **" {
                n148 = Index Array(array=w259) -> (element=w258:cluster{string[]})  [unwired: 1 in]
                n149 = call <vilib>:"NT Read String.vi"("Name"=w261) -> ("String"=w260:string)  [unwired: 9 in, 1 out]
                n150 = Unbundle(w258) -> (w256:string[])
                n151 = Match First String(2:w256, 3:w260) -> (0:w257:i32)  [unwired: 1 out]
                n152 = property on="Test Ring" class="Ring (strict)"("Value"=w257, "Strings []"=w256) -> ()  [unwired: 2 in, 2 out]
                n153 = property on="Test Ring" class="Ring (strict)"("Visible"=TRUE) -> ()  [unwired: 2 in, 2 out]
                n154 = property on="Test Slider" class="Slide (strict)"("Visible"=FALSE) -> ()  [unwired: 2 in, 2 out]
              }
              frame "White Balance  **" {
                n155 = Index Array(array=w267, index=1) -> (element=w268:cluster{string[]})
                n156 = call <vilib>:"NT Read String.vi"("Name"=w270) -> ("String"=w269:string)  [unwired: 9 in, 1 out]
                n157 = Unbundle(w268) -> (w265:string[])
                n158 = Match First String(2:w265, 3:w269) -> (0:w264:i32)  [unwired: 1 out]
                n159 = property on="Test Ring" class="Ring (strict)"("Value"=w264, "Strings []"=w265) -> ()  [unwired: 2 in, 2 out]
                n160 = property on="Test Ring" class="Ring (strict)"("Visible"=TRUE) -> ()  [unwired: 2 in, 2 out]
                n161 = property on="Test Slider" class="Slide (strict)"("Visible"=FALSE) -> ()  [unwired: 2 in, 2 out]
              }
              frame "Exposure  **" {
                n162 = Index Array(array=w276, index=2) -> (element=w277:cluster{string[]})
                n163 = call <vilib>:"NT Read String.vi"("Name"=w279) -> ("String"=w278:string)  [unwired: 9 in, 1 out]
                n164 = Unbundle(w277) -> (w273:string[])
                n165 = Match First String(2:w273, 3:w278) -> (0:w274:i32)  [unwired: 1 out]
                n166 = property on="Test Ring" class="Ring (strict)"("Value"=w274, "Strings []"=w273) -> ()  [unwired: 2 in, 2 out]
                n167 = property on="Test Ring" class="Ring (strict)"("Visible"=TRUE) -> ()  [unwired: 2 in, 2 out]
                n168 = property on="Test Slider" class="Slide (strict)"("Visible"=FALSE) -> ()  [unwired: 2 in, 2 out]
              }
              frame "Exposure Priority  **" {
                n169 = Index Array(array=w285, index=3) -> (element=w286:cluster{string[]})
                n170 = call <vilib>:"NT Read String.vi"("Name"=w288) -> ("String"=w287:string)  [unwired: 9 in, 1 out]
                n171 = Unbundle(w286) -> (w282:string[])
                n172 = Match First String(2:w282, 3:w287) -> (0:w283:i32)  [unwired: 1 out]
                n173 = property on="Test Ring" class="Ring (strict)"("Value"=w283, "Strings []"=w282) -> ()  [unwired: 2 in, 2 out]
                n174 = property on="Test Ring" class="Ring (strict)"("Visible"=TRUE) -> ()  [unwired: 2 in, 2 out]
                n175 = property on="Test Slider" class="Slide (strict)"("Visible"=FALSE) -> ()  [unwired: 2 in, 2 out]
              }
              frame "Color Enable  **" {
                n176 = Index Array(array=w294, index=4) -> (element=w295:cluster{string[]})
                n177 = call <vilib>:"NT Read String.vi"("Name"=w297) -> ("String"=w296:string)  [unwired: 9 in, 1 out]
                n178 = Unbundle(w295) -> (w291:string[])
                n179 = Match First String(2:w291, 3:w296) -> (0:w292:i32)  [unwired: 1 out]
                n180 = property on="Test Ring" class="Ring (strict)"("Value"=w292, "Strings []"=w291) -> ()  [unwired: 2 in, 2 out]
                n181 = property on="Test Ring" class="Ring (strict)"("Visible"=TRUE) -> ()  [unwired: 2 in, 2 out]
                n182 = property on="Test Slider" class="Slide (strict)"("Visible"=FALSE) -> ()  [unwired: 2 in, 2 out]
              }
              frame Default {
                n183 = property on="Test Ring" class="Ring (strict)"("Visible"=FALSE) -> ()  [unwired: 2 in, 2 out]
                n184 = property on="Test Slider" class="Slide (strict)"("Visible"=FALSE) -> ()  [unwired: 2 in, 2 out]
              }
              frame "Brightness  **", "Color Level  **", "Compression  **", "FPS  **", "Sharpness  **" {
                n185 = call <vilib>:"NT Read Number.vi"("Name"=w303) -> ("Numeric"=w302:dbl)  [unwired: 9 in, 1 out]
                n186 = local write "Test Slider"(w302) -> ()
                n187 = property on="Test Slider" class="Slide (strict)"("Visible"=TRUE, "Scale.Maximum"=100.0 ("Scale.Range:Maximum")) -> ()  [unwired: 2 in, 2 out]
                n188 = property on="Test Ring" class="Ring (strict)"("Visible"=FALSE) -> ()  [unwired: 2 in, 2 out]
              }
            }
          }
        }
        n189 = property on="Progress" class="Clust (strict)"("Visible"=FALSE) -> ()  [unwired: 2 in, 2 out]
      }
      event "Test Name": Mouse Enter {
        # "Populate the ring with the list of tests"
        n190 = event-data() -> ()  [unwired: 1 in, 1 out]
        n191 = call <vilib>:"NT Read String Array.vi"("Name"="/TestMode/TestList") -> ("String Array"=w312:string[])  [unwired: 9 in, 1 out]
        n192 = Build Array (concatenate)("Select the test to run...", w312) -> (w311:string[])
        n193 = property on="Test Name" class="Ring (strict)"("Strings []"=w311) -> ()  [unwired: 2 in, 2 out]
      }
      event "Test Name": Value Change {
        w315 = FALSE ("Visible")
        # "Tell the robot the test name to run"
        n194 = event-data() -> ("NewVal"=w319:u16)  [unwired: 1 in]
        n195 = property on="Test Name" class="Ring (strict)"() -> ("Strings []"=w320:string[])  [unwired: 2 in, 2 out]
        n196 = local write "Progress"(T7 {"Test Progress"=0, "Test Progress Text"=""} ("Progress")) -> ()
        n197 = Index Array(array=w320, index=w319) -> (element=w318:string)
        n198 = call <vilib>:"NT Write String.vi"("String"=w318, "Name"="/TestMode/TestName") -> ()  [unwired: 9 in, 1 out]
        n199 = property on="Progress" class="Clust (strict)"("Visible"=TRUE) -> ()  [unwired: 2 in, 2 out]
        n200 = property on="Motor" class="Clust (strict)"("Visible"=w315) -> ()  [unwired: 2 in, 2 out]
        n201 = property on="Test Slider" class="Slide (strict)"("Visible"=w315) -> ()  [unwired: 2 in, 2 out]
        n202 = property on="On/Off" class="Bool (strict)"("Visible"=w315) -> ()  [unwired: 2 in, 2 out]
        n203 = property on="Rev/Fwd" class="Clust (strict)"("Visible"=w315) -> ()  [unwired: 2 in, 2 out]
        n204 = property on="Test Ring" class="Ring (strict)"("Visible"=w315) -> ()  [unwired: 2 in, 2 out]
      }
      event "Command Selection": Value Change {
        # "Get the params and show in table"
        n205 = event-data() -> ("NewVal"=w325:i32)  [unwired: 1 in]
        n206 = property on="Command Selection" class="MCListbox (strict)"() -> ("ItemNames"=w323:string[][])  [unwired: 2 in, 2 out]
        n207 = call <vilib>:"WPI_DashboardUpdate Command Params.vi"("NewVal"=w325, "Commands"=w323, "Param Tbl"=w324) -> ()  [unwired: 8 in, 1 out]
      }
      event "Execute Command": Value Change {
        # "Started one, Unique ID holds\nresponse"
        n208 = event-data() -> ()  [unwired: 1 in, 1 out]
        n209 = property on="Command Selection" class="MCListbox (strict)"() -> ("ItemNames"=w337:string[][])  [unwired: 2 in, 2 out]
        n210 = Index Array(array=w337, index (row)="Command Selection", index (col)=0) -> (element=w335:string)
        n211 = call <vilib>:"Invoke Commands.vi"("Command Params"="Command Params", "Function Name"=w335) -> ("Params"=w331:u8, "Started"=w330:bool)  [unwired: 7 in, 1 out]
        n212 = Array Subset(array="Command Params", length (row)=w331) -> (w332:string[][])  [unwired: 3 in]
        n213 = Select(t="Executing" ("Cmd Status"), s=w330, f="" ("Cmd Status")) -> (s? t:f=→"Cmd Status":string)
      }
      event "Command Selection": Double Click {
        n214 = event-data() -> ("Row"=w347:i32)  [unwired: 1 in]
        n215 = property on="Command Selection" class="MCListbox (strict)"() -> ("ItemNames"=w350:string[][])  [unwired: 2 in, 2 out]
        n216 = local read "Command Params"() -> (w345:string[][])
        n217 = Index Array(array=w350, index (row)=w347, index (col)=0) -> (element=w348:string)
        n218 = call <vilib>:"Invoke Commands.vi"("Command Params"=w345, "Function Name"=w348) -> ("Params"=w344:u8, "Started"=w339:bool)  [unwired: 7 in, 1 out]
        n219 = Array Subset(array=w345, length (row)=w344) -> (w343:string[][])  [unwired: 3 in]
        n220 = Select(t="Executing" ("Cmd Status"), s=w339, f="" ("Cmd Status")) -> (s? t:f=w340:string)
        n221 = local write "Cmd Status"(w340) -> ()
      }
      event "CheckList": Double Click {
        # "Shift clears all"
        # "Update symbols on the listbox"
        n222 = event-data() -> ("PlatMods.Shift"=w353:bool, "Row"=w355:i32)  [unwired: 1 in]
        n223 = case shown="True" w353 {
          tunnel: w355 -> [w359 _]
          tunnel: 1 -> [w358 _]
          frame False {
            n224 = property on="CheckList" class="LstBox (strict)"() -> ("Item Symbols"=w357:i32[])  [unwired: 2 in, 2 out]
            n225 = Replace Array Subset(array=w357, new element=w358, index=w359) -> (w356:i32[])
            n226 = property on="CheckList" class="LstBox (strict)"("Item Symbols"=w356) -> ()  [unwired: 2 in, 2 out]
          }
          frame True {
            w360 = 0 ("Top Row")
            n227 = property on="CheckList" class="LstBox (strict)"() -> ("Number of Rows"=w362:u32)  [unwired: 2 in, 2 out]
            n228 = Initialize Array(0, w362) -> (w361:i32[])
            n229 = property on="CheckList" class="LstBox (strict)"("Top Row"=w360, "Value"=w360, "Item Symbols"=w361) -> ()  [unwired: 2 in, 2 out]
          }
        }
      }
      event "CheckList": Key Down {
        # "Update symbols on the listbox\nLeft and right keys check and uncheck"
        n230 = event-data() -> ("VKey"=w367:T22)  [unwired: 1 in]
        n231 = case shown="\"Left\", \"Right\"" w367 {
          selector: w367 -> [w372 _]
          tunnel: eventvkey."Left" ("VKey") -> [w370 _]
          frame "Left", "Right" {
            n232 = Equal?(x=w370, y=w372) -> (x = y?=w371:bool)
            n233 = Select(t=0, s=w371, f=1) -> (s? t:f=w373:i32)
            n234 = property on="CheckList" class="LstBox (strict)"() -> ("Item Symbols"=w376:i32[])  [unwired: 2 in, 2 out]
            n235 = Replace Array Subset(array=w376, new element=w373, index="CheckList") -> (w375:i32[])
            n236 = property on="CheckList" class="LstBox (strict)"("Item Symbols"=w375) -> ()  [unwired: 2 in, 2 out]
          }
          frame Default {
          }
        }
      }
      event "DB Camera Config": Value Change {
        # "Show or hide the cluster of controls, store in ini file"
        n237 = event-data() -> ("NewVal"=w381:bool)  [unwired: 1 in]
        n238 = case shown="False" w381 {
          tunnel: w380 -> [w390 _]
          tunnel: [w383 w401] -> w379
          tunnel: w378 -> [w382 w401]
          frame False {
            w397 = "Camera"
            w400 = FALSE ("Visible")
            n239 = local read "Camera Settings"() -> (w389:T2)
            n240 = Index Array(array=w390) -> (element=w393:cluster{string[]})  [unwired: 1 in]
            n241 = Unbundle(w389) -> ("Frame Rate"=w388:i32, "Compression"=w387:i32, "Size"=w391:u16)
            n242 = Unbundle(w393) -> (w392:string[])
            n243 = Index Array(array=w392, index=w391) -> (element=w386:string)
            n244 = call-poly <vilib>:"Write Key.vi"("section"=w397, "value"=w386, "key"="Size", "refnum"=w382) -> ("refnum out"=w399:T20)  [unwired: 2 in, 5 out]
            n245 = call-poly <vilib>:"Write Key.vi"("section"=w397, "value"=w388, "key"="FrameRate", "refnum"=w399) -> ("refnum out"=w398:T20)  [unwired: 1 in, 6 out]
            n246 = property on="Camera Settings" class="Clust (strict)"("Visible"=w400) -> ()  [unwired: 2 in, 2 out]
            n247 = local write "DB Camera Config"(w400) -> ()
            n248 = call-poly <vilib>:"Write Key.vi"("section"=w397, "value"=w387, "key"="Compression", "refnum"=w398) -> ("refnum out"=w384:T20)  [unwired: 1 in, 6 out]
            n249 = call <vilib>:"Close Config Data.vi"("refnum"=w384) -> ("file path"=w385:path)  [unwired: 2 in, 8 out]
            n250 = call <vilib>:"Open Config Data.vi"("configuration file path"=w385) -> ("refnum"=w383:T20)  [unwired: 8 in, 2 out]
          }
          frame True {
            n251 = property on="Camera Settings" class="Clust (strict)"("Visible"=TRUE) -> ()  [unwired: 2 in, 2 out]
          }
        }
      }
      event "Camera Settings": Value Change {
        # "Update summary string when any elements of DB camera change"
        n252 = event-data() -> ("NewVal"=w415:T2)  [unwired: 1 in]
        n253 = Index Array(array=w411) -> (element=w410:cluster{string[]})  [unwired: 1 in]
        n254 = Unbundle(w415) -> ("Frame Rate"=w406:i32, "Compression"=w405:i32, "Size"=w408:u16)
        n255 = Unbundle(w410) -> (w409:string[])
        n256 = Index Array(array=w409, index=w408) -> (element=w407:string)
        n257 = Format Into String(format string="%s   %dfps   %d%%", w407, w406, w405) -> (resulting string=w412:string)  [unwired: 2 in, 1 out]
        n258 = Build Array(w412) -> (w413:string[])
        n259 = property on="DB Camera Config" class="Bool (strict)"("Strings [4]"=w413) -> ()  [unwired: 2 in, 2 out]
      }
      event "Motor.Enable": Value Change {
        # "When the test mode otor enable helper is set, update that\ntree row item's value"
        n260 = event-data() -> ("NewVal"=w422:bool)  [unwired: 1 in]
        n261 = Unbundle("Motor") -> ("Value"=w421:dbl)  [unwired: 1 out]
        n262 = Select(t=w421, s=w422, f=0.0) -> (s? t:f=w419:dbl)
        n263 = call <vilib>:"NT Write Number.vi"("Numeric"=w419, "Name"=w418) -> ()  [unwired: 9 in, 1 out]
      }
      event "Test Slider": Value Change {
        # "When the test mode slider helper is set, update that\ntree row item's value"
        n264 = event-data() -> ("NewVal"=w426:dbl)  [unwired: 1 in]
        n265 = call <vilib>:"NT Write Number.vi"("Numeric"=w426, "Name"=w427) -> ()  [unwired: 9 in, 1 out]
      }
      event "On/Off": Value Change {
        # "When the test mode on/off helper value is set, update that\ntree row item's value"
        n266 = event-data() -> ("NewVal"=w432:bool)  [unwired: 1 in]
        n267 = Boolean To (0,1)(Boolean=w432) -> (0, 1=w431:i16)
        n268 = call <vilib>:"NT Write Number.vi"("Numeric"=w431, "Name"=w430) -> ()  [unwired: 9 in, 1 out]
      }
      event "Rev/Fwd": Value Change {
        # "When the test mode helper value for relays is set, update that\ntree row item's value"
        n269 = event-data() -> ("NewVal.Forward"=w441:bool, "NewVal.Reverse"=w440:bool)  [unwired: 1 in]
        n270 = Boolean To (0,1)(Boolean=w441) -> (0, 1=w437:i16)
        n271 = Boolean To (0,1)(Boolean=w440) -> (0, 1=w439:i16)
        n272 = Negate(x=w439) -> (-x=w438:i16)
        n273 = Add(x=w437, y=w438) -> (x+y=w436:i16)
        n274 = call <vilib>:"NT Write Number.vi"("Numeric"=w436, "Name"=w435) -> ()  [unwired: 9 in, 1 out]
      }
      event "Test Ring": Value Change {
        # "When a test mode helper value is selected from the ring,\nset the tree item's variable to the string value"
        n275 = event-data() -> ("NewVal"=w446:u16)  [unwired: 1 in]
        n276 = property on="Test Ring" class="Ring (strict)"() -> ("Strings []"=w447:string[])  [unwired: 2 in, 2 out]
        n277 = Index Array(array=w447, index=w446) -> (element=w445:string)
        n278 = call <vilib>:"NT Write String.vi"("String"=w445, "Name"=w444) -> ()  [unwired: 9 in, 1 out]
      }
      event "Rec Mode": Value Change {
        # "Update globals for recording mode and path to read log from.\nClear when logging and let NetworkTables set path for vision to\nuse."
        n279 = event-data() -> ("NewVal"=w459:enum32{"Stop", "Record", "Playback"})  [unwired: 1 in]
        n280 = global write "WPI_DashboardLogging Global.vi" "Logging Filename"(path "") -> ()
        n281 = global write "WPI_DashboardLogging Global.vi" "Recording"(w459) -> ()
        n282 = case shown="\"Playback\"" w459 {
          tunnel: w458 -> [_ w461 w470]
          tunnel: [_ _ w469] -> w455
          tunnel: [_ _ w468] -> _
          tunnel: w453 -> [_ _ w466]
          tunnel: cluster{i32, i32} {-250, 170} -> [_ _ w465]
          tunnel: [_ _ T23 {"Image Size"=TRUE, "Image Type"=TRUE, "Pixel Value"=TRUE, "ROI Information"=TRUE, "Zoom Factor"=FALSE} ("Image Information Shown:All Elements")] -> w451
          tunnel: [_ _ TRUE ("Zoom Factor")] -> w450
          tunnel: w449 -> [_ _ w462]
          frame Default {
          }
          frame "Stop", "Record" {
            # "Place Window too"
            n283 = invoke class="VI" method="FP.Close"(reference=w461) -> (reference out=w460:refnum<vi>)  [unwired: 2 in, 2 out]
            n284 = invoke class="VI" method="Abort VI"(reference=w460) -> ()  [unwired: 2 in, 3 out]
          }
          frame "Playback" {
            n285 = call "Open Playback Panel.vi"("Offset"=w465, "DB VI Ref"=w466, "Playback in"=w470) -> ("Playback out"=w467:refnum<vi>)  [unwired: 8 in]
            n286 = register-events(w467, w462) -> (reference out=w469:refnum<event-registration>, error out=w468:errorcluster)  [unwired: 2 in]
          }
        }
        n287 = property on="Camera Image" class="ImageControl"("Image Information Shown"=w451, "Image Information Visible"=w450) -> ()  [unwired: 2 in, 2 out]
        n288 = call <vilib>:"WPI_DashboardNT Log FieldName Cache.vi"("Operation"=enum16{"Lookup/Add", "Index", "Clear"}."Clear") -> ()  [unwired: 8 in, 3 out]
      }
      event Panel Close {
        w472 = enum32{"Stop", "Record", "Playback"}."Stop" ("Rec Mode")
        # "Playback window has been closed, abort"
        n289 = event-data() -> ()  [unwired: 1 in, 4 out]
        n290 = local write "Rec Mode"(w472) -> ()
        n291 = global write "WPI_DashboardLogging Global.vi" "Recording"(w472) -> ()
      }
      event Panel Close {
        # "Abort playback window and ourself"
        n292 = event-data() -> ()  [unwired: 1 in, 4 out]
        n293 = invoke class="VI" method="FP.Close"(reference=w478) -> (reference out=w477:refnum<vi>)  [unwired: 2 in, 2 out]
        n294 = invoke class="VI" method="Abort VI"(reference=w477) -> (error out=w476:errorcluster)  [unwired: 2 in, 2 out]
        n295 = invoke class="VI" method="Abort VI"(error in=w476) -> ()  [unwired: 2 in, 3 out]
      }
      event User Event {
        n296 = event-data() -> ("IDs"=w486:cluster{"RPC field ID":u16, "Unique ID":u16}, "String"=w485:string)  [unwired: 1 in]
        n297 = Bundle("IDs"=w486, "String"=w485) -> (w484:T9)  [unwired: 1 in]
        n298 = call <vilib>:"Retrieve RPC Response.vi"("RPC Response"=w484) -> ("Output"=w481:string[][])  [unwired: 10 in]
        n299 = Build Array (concatenate)(w479, w481) -> (w480:string[][])
        n300 = local write "Command Params"(w480) -> ()
        n301 = local write "Cmd Status"("" ("Cmd Status")) -> ()
      }
      event "Vision": Value Change {
        # "Enable/Disable Compression slider.\nHW USB is hard-coded into the camera"
        n302 = event-data() -> ("NewVal"=w493:u16)  [unwired: 1 in]
        n303 = Equal?(x=w493, y=u32 2 ("milliseconds to wait")) -> (x = y?=w491:bool)
        n304 = Select(t=T24."Disabled and Grayed Out" ("Disabled"), s=w491, f=T24."Enabled" ("Disabled")) -> (s? t:f=w488:T24)
        n305 = property on="Compression" class="Slide (strict)"("DisabledEnum"=w488) -> ()  [unwired: 2 in, 2 out]
      }
    }
  }
  n306 = while {
    tunnel: w47 -> [w496]
    i -> [w499]
    stop <- FALSE stop-if-true
    n307 = Wait (ms)(milliseconds to wait=u32 100) -> ()  [unwired: 1 out]
    n308 = case shown="\"Playback\"" "Rec Mode" {
      tunnel: w499 -> [_ _ w514]
      tunnel: [u32 2829099 ("Base Color") u32 11141120 ("Target Color") w503] -> w495
      frame "Stop", Default {
        # "Reset the color, extra updates don't cost much"
      }
      frame "Record" {
      }
      frame "Playback" {
        # "Playback"
        n309 = Quotient & Remainder(x=w514, y=u32 50 ("milliseconds to wait")) -> (x-y*floor(x/y)=w510:u32)  [unwired: 1 out]
        n310 = Divide(x=w510, y=u32 50 ("milliseconds to wait")) -> (x/y=w507:dbl)
        n311 = Multiply(x=6.283185307179586, y=w507) -> (x*y=w512:dbl)
        n312 = Sine(x=w512) -> (sin(x)=w511:dbl)
        n313 = Absolute Value(x=w511) -> (abs(x)=w504:dbl)
        n314 = call "Interpolate RGB Color.vi"("Proportion"=w504, "Target Color"=u32 30976, "Base Color"=u32 2829099) -> ("Result Color"=w503:u32)  [unwired: 8 in]
      }
    }
    n315 = property class="Pane"(reference=w496, "PaneColor"=w495) -> ()  [unwired: 1 in, 2 out]
  }
  n316 = local write "Dashboard Tab"(T1."Drive" ("Dashboard Tab")) -> ()
  n317 = property on="On/Off" class="Bool (strict)"("Visible"=w15) -> ()  [unwired: 2 in, 2 out]
  n318 = property on="Motor" class="Clust (strict)"("Visible"=w15) -> ()  [unwired: 2 in, 2 out]
  n319 = property on="Progress" class="Clust (strict)"("Visible"=w15) -> ()  [unwired: 2 in, 2 out]
  n320 = property on="Test Ring" class="Ring (strict)"("Visible"=w15) -> ()  [unwired: 2 in, 2 out]
  n321 = property on="Rev/Fwd" class="Clust (strict)"("Visible"=w15) -> ()  [unwired: 2 in, 2 out]
  n322 = property on="Camera Settings" class="Clust (strict)"("Visible"=w15) -> ()  [unwired: 2 in, 2 out]
  n323 = while {
    tunnel: u16 1741 ("timeout ms (25000)") -> [w516]
    stop <- FALSE stop-if-true
    n324 = TCP Create Listener(10:w516) -> (0:w515:errorcluster, 3:w517:refnum<k5>)  [unwired: 4 in, 1 out]
    n325 = case shown="No Error" w515 {
      selector: w515 -> [w519 _]
      tunnel: w517 -> [w520 _]
      frame No Error {
        n326 = while {
          tunnel: w520 -> [w523]
          tunnel: w519 -> [w522]
          stop <- FALSE stop-if-true
          n327 = TCP Wait On Listener(8:w522, 11:w523) -> (0:w524:errorcluster, 4:w525:refnum<k5>)  [unwired: 2 in, 3 out]
          n328 = local write "TCP"(w525) -> ()
          n329 = case shown="No Error" w524 {
            frame No Error {
            }
            frame Error {
              n330 = Wait (ms)(milliseconds to wait=u32 1000) -> ()  [unwired: 1 out]
            }
          }
        }
      }
      frame Error {
        n331 = Wait (ms)(milliseconds to wait=u32 1000) -> ()  [unwired: 1 out]
      }
    }
  }
  n332 = local write "DB Camera Config"(w15) -> ()
  n333 = local write "Command Params"(string[][] [] ("Command Params")) -> ()
  n334 = global write "WPI_DashboardLogging Global.vi" "Recording"(w41) -> ()
  n335 = local write "Command Selection"(u16 0 ("milliseconds to wait")) -> ()
  n336 = local write "Rec Mode"(w41) -> ()
